vi "WPI_UltrasonicClose.vi"   [LabVIEW 2017]
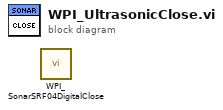
[diagram p0: block diagram]
diagram:
  n1 = call <vilib>:"WPI_SonarSRF04DigitalClose.vi"() -> ()  [unwired: 11 in, 1 out]
